vi "Drive main.vi"() -> ()   [LabVIEW 2018]
uses:
  <vilib>/Rock Robotics/WPI/ThirdParty/Phoenix-LabVIEW/Motor Controller/Controls/CTRE_Phoenix_MotorControl_ControlMode.ctl
  <vilib>/Rock Robotics/WPI/Solenoid/WPI_SolenoidValue.ctl
  <vilib>/Rock Robotics/WPI/ThirdParty/Phoenix-LabVIEW/Motor Controller/Get/CTRE_Phoenix_MotorController_GetSelectedSensorData.vi
  <vilib>/Rock Robotics/Network Tables/NT Write Number.vi
  Robot Global Data.vi
  <vilib>/Rock Robotics/WPI/Solenoid/WPI_SolenoidSetEnum.vi
panel:
  out "Right Encoder Pos":i32
  out "Left Encoder Pos":i32
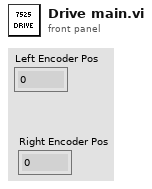
[diagram p1: front panel]
types:
  T1 = typedef "WPI_SolenoidValue.ctl" = enum16{"Off", "On", "Forward", "Reverse"}
  T2 = typedef "CTRE_Phoenix_MotorControl_ControlMode.ctl" = u16
  T3 = typedef "ElevatorAndShift2.ctl" = cluster{"Drive Shift":bool, "Ground":bool, "Hatch Low":bool, "Hatch Mid":bool, "Hatch High":bool, "Cargo Low":bool, "Cargo Mid":bool, "Cargo High":bool, "Cargo Ship":bool, "Cargo Feed":bool}
  T4 = typedef "WPI_SolenoidDevRef.ctl" = cluster{"DevStatus":errorcluster, "Pneumatics Control Module":u8, "Forward Solenoid Channel":T5, "Reverse Solenoid Channel":T5}
  T5 = typedef "WPI_SolenoidChannel.ctl" = enum8{"Solenoid 0", "Solenoid 1", "Solenoid 2", "Solenoid 3", "Solenoid 4", "Solenoid 5", "Solenoid 6", "Solenoid 7", "Invalid"}
  T6 = typedef "WPI_MotorControlDeviceRef.ctl" = cluster{"DeviceStatus":errorcluster, "Type":T7, "PWM":cluster{"PWM Channel":T8, "DeadBand":T9}, "CAN":cluster{"Device Number":u8, "SetOutput VI Ref":variant, "GetOutput VI Ref":variant, "Enable VI Ref":variant, "Disable VI Ref":variant, "Data":variant}, "Invert":bool, "DIO PWM":cluster{"PWM \"Enable\" Channel":T8, "DIOChannel":T10, "PWM Rate":dbl}}
  T7 = typedef "WPI_MotorControlType.ctl" = enum16{"PWM", "CAN", "DIO PWM"}
  T8 = typedef "FPGA_DIOPWMChannel.ctl" = enum8{"PWM 0", "PWM 1", "PWM 2", "PWM 3", "PWM 4", "PWM 5", "PWM 6", "PWM 7", "PWM 8", "PWM 9", "PWM MXP 0", "PWM MXP 1", "PWM MXP 2", "PWM MXP 3", "PWM MXP 4", "PWM MXP 5", "PWM MXP 6", "PWM MXP 7", "PWM MXP 8", "PWM MXP 9", "Invalid"}
  T9 = typedef "WPI_PWMDeadband.ctl" = cluster{"Name":string, "maxPositivePwm":i32, "minPositivePwm":i32, "centerPwm":i32, "maxNegativePwm":i32, "minNegativePwm":i32, "angularRange":u16}
  T10 = typedef "FPGA_DIOChannel.ctl" = enum8{"DIO 0", "DIO 1", "DIO 2", "DIO 3", "DIO 4", "DIO 5", "DIO 6", "DIO 7", "DIO 8", "DIO 9", "DIO MXP 0", "DIO MXP 1", "DIO MXP 2", "DIO MXP 3", "DIO MXP 4", "DIO MXP 5", "DIO MXP 6", "DIO MXP 7", "DIO MXP 8", "DIO MXP 9", "DIO MXP 10", "DIO MXP 11", "DIO MXP 12", "DIO MXP 13", "DIO MXP 14", "DIO MXP 15", "SPI Port CS1", "SPI Port CS2", "SPI Port CS3", "SPI Port MISO", "SPI Port MOSI", "Invalid"}
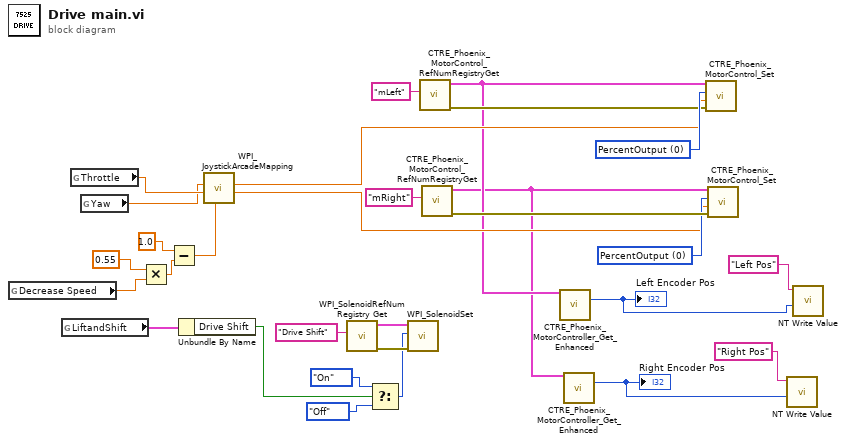
[diagram p0: block diagram]
diagram:
  w24 = T2 0 items=["PercentOutput"=0, "Position"=1, "Velocity"=2, "Current"=3, "Follower"=5, "MotionProfile"=6, "MotionMagic"=7, "MotionProfileArc"=10, "Disabled"=15] ("Control Mode")
  w29 = T2 0 items=["PercentOutput"=0, "Position"=1, "Velocity"=2, "Current"=3, "Follower"=5, "MotionProfile"=6, "MotionMagic"=7, "MotionProfileArc"=10, "Disabled"=15] ("Control Mode")
  n1 = global read "Robot Global Data.vi" "Decrease Speed"() -> (w7:dbl)
  n2 = global read "Robot Global Data.vi" "LiftandShift"() -> (w21:T3)
  n3 = global read "Robot Global Data.vi" "Throttle"() -> (w13:dbl)
  n4 = global read "Robot Global Data.vi" "Yaw"() -> (w12:dbl)
  n5 = Multiply(x=0.55, y=w7) -> (x*y=w9:dbl)
  n6 = Subtract(x=1.0, y=w9) -> (x-y=w8:dbl)
  n7 = Unbundle By Name(w21) -> ("Drive Shift"=w16:bool)
  n8 = call <vilib>:"WPI_JoystickArcadeMapping.vi"("Max Output"=w8, "Y axis value"=w13, "X axis value"=w12) -> ("Right Motor Value"=w22:dbl, "Left Motor Value"=w23:dbl)  [unwired: 7 in]
  n9 = call <vilib>:"WPI_SolenoidRefNum Registry Get.vi"("refnum name"="Drive Shift") -> ("error out"=w20:errorcluster, "SolenoidDevRef"=w19:T4)  [unwired: 9 in]
  n10 = Select(t=WPI_SolenoidValue."On" ("Value"), s=w16, f=WPI_SolenoidValue."Off" ("Value")) -> (s? t:f=w15:T1)
  n11 = call-poly <vilib>:"WPI_SolenoidSet.vi"("error in (no error)"=w20, "Value"=w15, "SolenoidDevRef"=w19) -> ()  [unwired: 7 in, 2 out]
  n12 = call <vilib>:"CTRE_Phoenix_MotorControl_RefNumRegistryGet.vi"("refnum name"="mLeft") -> ("error out"=w28:errorcluster, "PhoenixMotorControlDevRef"=w6:T6)  [unwired: 9 in]
  n13 = call <vilib>:"CTRE_Phoenix_MotorControl_RefNumRegistryGet.vi"("refnum name"="mRight") -> ("error out"=w25:errorcluster, "PhoenixMotorControlDevRef"=w5:T6)  [unwired: 9 in]
  n14 = call-poly <vilib>:"CTRE_Phoenix_MotorController_Get_Enhanced.vi"("PhoenixMotorControlDevRef"=w6) -> ("Position (Raw Sensor Units)"=w3:i32)  [unwired: 11 in, 3 out]
  "Left Encoder Pos" <- w3
  n15 = call-poly <vilib>:"CTRE_Phoenix_MotorController_Get_Enhanced.vi"("PhoenixMotorControlDevRef"=w5) -> ("Position (Raw Sensor Units)"=w4:i32)  [unwired: 11 in, 3 out]
  "Right Encoder Pos" <- w4
  n16 = call <vilib>:"CTRE_Phoenix_MotorControl_Set.vi"("error in (no error)"=w28, "Output"=w23, "Control Mode"=w29, "PhoenixMotorControlDevRef"=w6) -> ()  [unwired: 6 in, 2 out]
  n17 = call <vilib>:"CTRE_Phoenix_MotorControl_Set.vi"("error in (no error)"=w25, "Output"=w22, "Control Mode"=w24, "PhoenixMotorControlDevRef"=w5) -> ()  [unwired: 6 in, 2 out]
  n18 = call-poly <vilib>:"NT Write Value.vi"("Numeric"=w4, "Name"="Right Pos") -> ()  [unwired: 9 in, 1 out]
  n19 = call-poly <vilib>:"NT Write Value.vi"("Numeric"=w3, "Name"="Left Pos") -> ()  [unwired: 9 in, 1 out]
